vi "LV SCISDK Get Parameter Double.vi"(8 "error in (no error)":errorcluster, 10 "handle":u64, 11 "Path":string) -> (0 "error out":errorcluster, 1 "function return":i32, 2 "handle out":u64, 3 "value":dbl)   [LabVIEW 2021, in "SciSDK_Labview.lvlib"]
doc: "SCISDKLABVIEW_DLL_API int LV_SCISDK_GetParameterDouble(char* Path, double* value, void* handle);"
uses:
  SciSDK_Labview.lvlib
  SciSDK_VC++/x64/Debug/SciSDK_Labview.dll
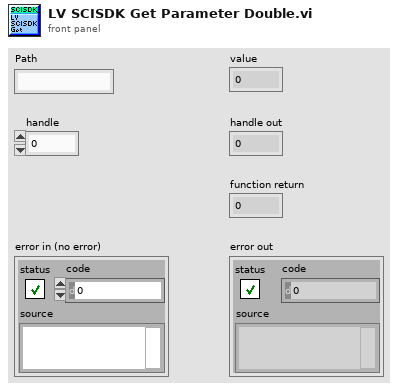
[diagram p1: front panel]
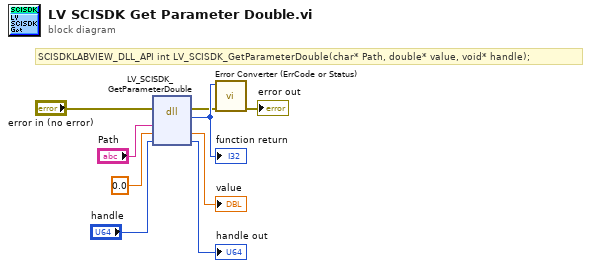
[diagram p0: block diagram]
diagram:
  # "SCISDKLABVIEW_DLL_API int LV_SCISDK_GetParameterDouble(char* Path, double* value, void* handle);"
  n1 = dll-call lib="C:/git/scisdk/SciSDK_VC++/x64/Debug/SciSDK_Labview.dll" fn="LV_SCISDK_GetParameterDouble"(error in="error in (no error)", "Path"="Path", "value"=0.0, "handle"="handle") -> (error out=w2:errorcluster, "return type"=w9:i32, "value"=→"value":dbl, "handle"=→"handle out":u64)  [unwired: 3 in, 1 out]
  "function return" <- w9
  n2 = call <userlib>:"Error Converter (ErrCode or Status).vi"("error in (no error)"=w2, "error code"=w9) -> ("error out"=→"error out":errorcluster)  [unwired: 9 in]
